vi "DHE_GetHardSemaphore.vi"(2 "timeout":i32=8000, 3 "error in (no error)":errorcluster) -> (7 "timed out":bool, 9 "error out":errorcluster)   [LabVIEW 2016]
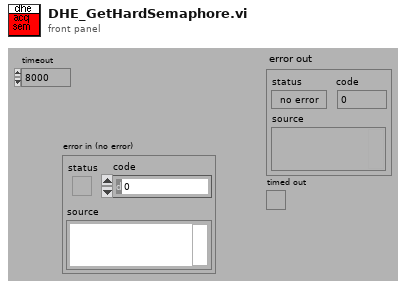
[diagram p1: front panel]
types:
  T1 = typedef "Semaphore RefNum" = refnum<k1>
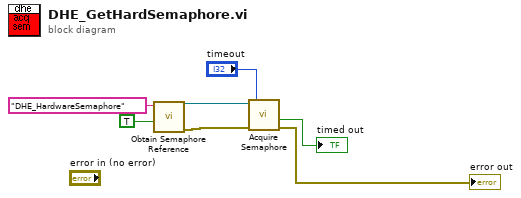
[diagram p0: block diagram]
diagram:
  n1 = call <vilib>:"Obtain Semaphore Reference.vi"("create if not found (T)"=TRUE, "name (unnamed)"="DHE_HardwareSemaphore") -> ("error out"=w5:errorcluster, "semaphore"=w4:T1)  [unwired: 2 in, 2 out]
  n2 = call <vilib>:"Acquire Semaphore.vi"("error in (no error)"=w5, "ms timeout (-1)"="timeout", "semaphore"=w4) -> ("error out"=→"error out":errorcluster, "timed out"=→"timed out":bool)  [unwired: 3 out]
